vi "_Main.vi"   [LabVIEW 2017, in "Joystick.lvlib"]
uses:
  Joystick.lvlib
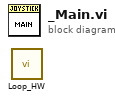
[diagram p0: block diagram]
diagram:
  n1 = call "Loop_HW.vi"() -> ()  [unwired: 12 in]
